vi "Initialization VI.vi"(8 "error in (no error)":errorcluster, 10 "Custom XML":string, 11 "Device Item Ref in":T1 format="%.0x") -> (0 "error out":errorcluster, 3 "Device Item Ref out":T1 format="%.0x")   [LabVIEW 2018, in "CAN Gateway System Explorer.lvlib"]
uses:
  CAN Gateway System Explorer.lvlib
  <vilib>/NI Veristand/Custom Device API/Custom Device Item Ref.ctl
  <vilib>/NI Veristand/Custom Device API/Custom Device API.lvlib
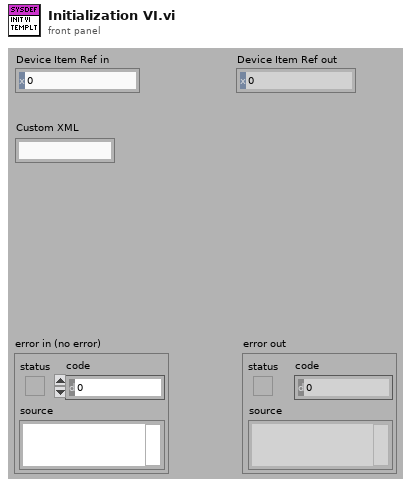
[diagram p1: front panel]
types:
  T1 = typedef "Custom Device API.lvlib/Custom Device Item Ref.ctl" = u64
  T2 = typedef "CAN Gateway System Explorer.lvlib/Alias DB data.ctl" = cluster{"Alias":string, "selected path":path}
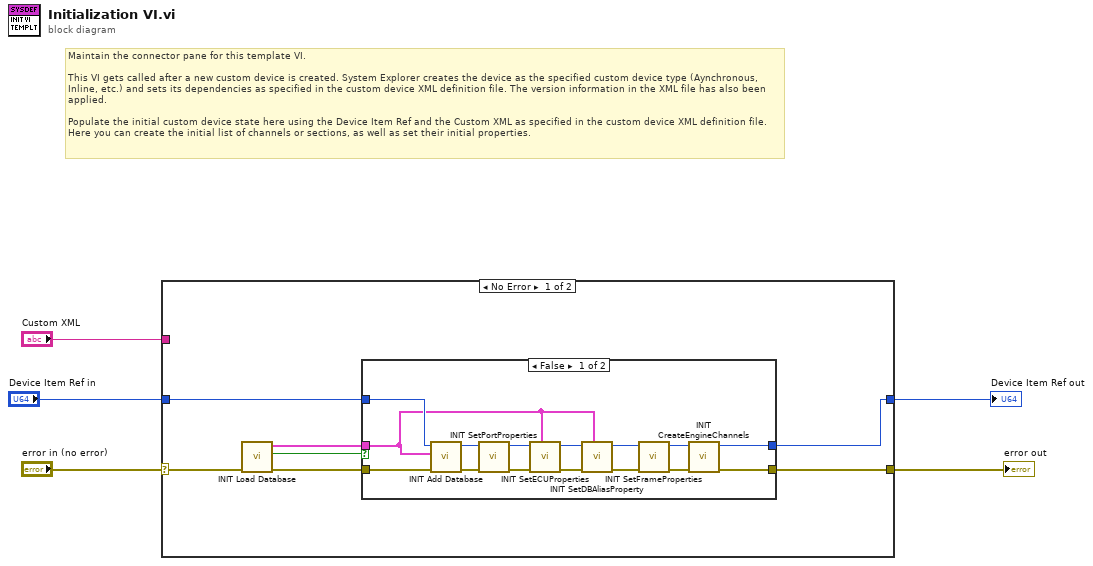
[diagram p0: block diagram]
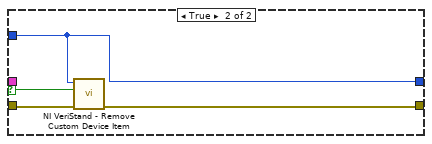
[diagram p2: hidden frame]
diagram:
  # "Maintain the connector pane for this template VI.\n\nThis VI gets called after a new custom device is created. System Explorer creates the device as the specified custom device type (Aynchronous, Inline, etc.) and sets its dependencies as specified in the custom device XML definition file. The version information in the XML file has also been applied.\n\nPopulate the initial custom device state here using the Device Item Ref and the Custom XML as specified in the custom device XML definition file. Here you can create the initial list of channels or sections, as well as set their initial properties."
  n1 = case shown="No Error" "error in (no error)" {
    selector: "error in (no error)" -> [w12 w33]
    tunnel: [w6 w33] -> w5
    tunnel: [w7 w32] -> w3
    tunnel: "Device Item Ref in" -> [w9 w32]
    tunnel: "Custom XML" -> [_ _]
    frame No Error {
      n2 = call "INIT Load Database.vi"("error in (no error)"=w12) -> ("error out"=w10:errorcluster, "cancelled"=w11:bool, "DB Alias data"=w8:T2)  [unwired: 8 in]
      n3 = case shown="False" w11 {
        selector: w11 -> [_ w30]
        tunnel: w10 -> [w27 w31]
        tunnel: w9 -> [w26 w29]
        tunnel: w8 -> [w13 _]
        tunnel: [w17 w29] -> w7
        tunnel: [w14 w28] -> w6
        frame False {
          n4 = call "INIT Add Database.vi"("error in (no error)"=w27, "DB Alias data"=w13, "Device Item Ref in"=w26) -> ("error out"=w16:errorcluster, "Device Item Ref out"=w15:T1)  [unwired: 7 in]
          n5 = call "INIT SetPortProperties.vi"("error in (no error)"=w16, "Device Item Ref in"=w15) -> ("error out"=w18:errorcluster, "Device Item Ref out"=w19:T1)  [unwired: 8 in]
          n6 = call "INIT SetECUProperties.vi"("DB Alias data"=w13, "error in (no error)"=w18, "Device Item Ref in"=w19) -> ("error out"=w20:errorcluster, "Device Item Ref out"=w21:T1)  [unwired: 7 in]
          n7 = call "INIT SetDBAliasProperty.vi"("DB Alias data"=w13, "error in (no error)"=w20, "Device Item Ref in"=w21) -> ("error out"=w22:errorcluster, "Device Item Ref out"=w23:T1)  [unwired: 7 in]
          n8 = call "INIT SetFrameProperties.vi"("error in (no error)"=w22, "Device Item Ref in"=w23) -> ("error out"=w24:errorcluster, "Device Item Ref out"=w25:T1)  [unwired: 8 in]
          n9 = call "INIT CreateEngineChannels.vi"("error in (no error)"=w24, "Device Item Ref in"=w25) -> ("error out"=w14:errorcluster, "Device Item Ref out"=w17:T1)  [unwired: 8 in]
        }
        frame True {
          n10 = call <vilib>:"NI VeriStand - Remove Custom Device Item.vi"("error in (no error)"=w31, "Force Delete (F)"=w30, "Item Ref in"=w29) -> ("error out"=w28:errorcluster)  [unwired: 7 in, 1 out]
        }
      }
    }
    frame Error {
    }
  }
  "error out" <- w5
  "Device Item Ref out" <- w3
